vi "Generate Simulated Data.vi"(7 "error in (no error)":cluster{"状态":bool, "代码":i32, "源":string} caption="错误输入（无错误）", 10 "信号类型":T1) -> (0 "error out":cluster{"状态":bool, "代码":i32, "源":string} caption="错误输出", 2 "图形数据":waveform(dbl)[](array[waveform]))   [LabVIEW 2012, in "Acquisition.lvlib"]
doc: "按硬件配置输入中的信号类型，生成采样波形。"
uses:
  Acquisition.lvlib
  Signal Type.ctl
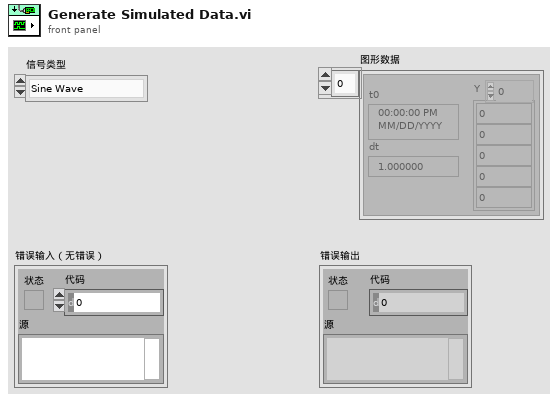
[diagram p1: front panel]
types:
  T1 = typedef "Acquisition.lvlib/Signal Type.ctl" = enum16{"Sine Wave", "Square with Noise"}
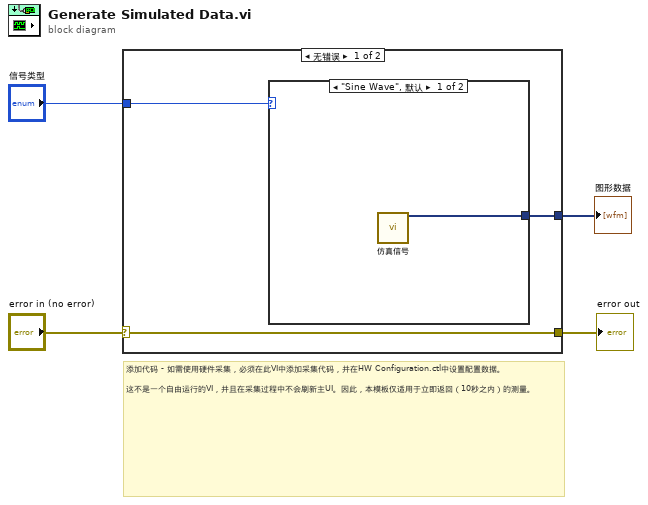
[diagram p0: block diagram]
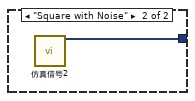
[diagram p2: hidden frame]
diagram:
  # "添加代码 - 如需使用硬件采集，必须在此VI中添加采集代码，并在HW Configuration.ctl中设置配置数据。\n\n这不是一个自由运行的VI，并且在采集过程中不会刷新主UI。因此，本模板仅适用于立即返回（10秒之内）的测量。"
  n1 = case shown="无错误" "error in (no error)" {
    selector: "error in (no error)" -> [w7 w10]
    tunnel: [w7 w10] -> w3
    tunnel: [w6 _] -> w2
    tunnel: "信号类型" -> [w5 _]
    frame No Error {
      n2 = case shown="\"Sine Wave\", 默认" w5 {
        tunnel: [w8 w9] -> w6
        frame "Sine Wave", Default {
          n3 = call "仿真信号"() -> ("Sine"=w8:dynamicdata)  [unwired: 14 in, 1 out]
        }
        frame "Square with Noise" {
          n4 = call "仿真信号2"() -> ("Square with Noise"=w9:dynamicdata)  [unwired: 14 in, 1 out]
        }
      }
    }
    frame Error {
    }
  }
  "error out" <- w3
  "图形数据" <- w2
